vi "Unflatten U16.vi"(3 "Flat Data":u8[](array[numeric]) format="%.0x", 4 "Endian":T1) -> (5 "U16":u16)   [LabVIEW 2021, in "DataTypes_CIF_U.lvlib"]
uses:
  DataTypes_CIF_U.lvlib
  Typedef/Endian.ctl
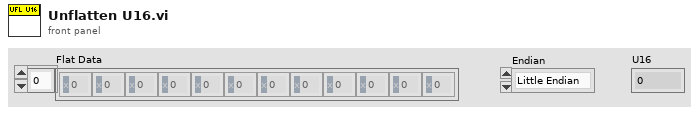
[diagram p1: front panel]
types:
  T1 = typedef "DataTypes_CIF_U.lvlib/Endian.ctl" = enum16{"Little Endian", "Big Endian"}
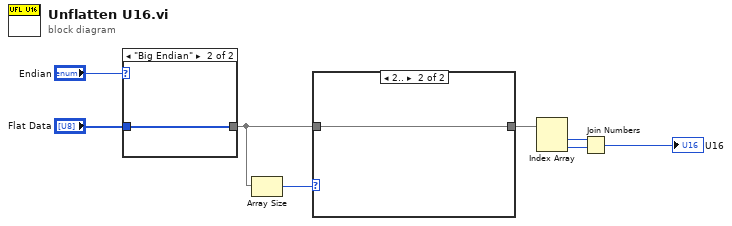
[diagram p0: block diagram]
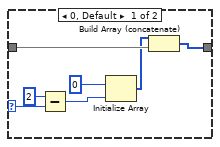
[diagram p2: hidden frame]
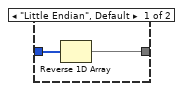
[diagram p3: hidden frame]
diagram:
  n1 = case shown="\"Big Endian\"" "Endian" {
    tunnel: "Flat Data" -> [w10 w11]
    tunnel: [w9 w11] -> w2
    frame "Little Endian", Default {
      n2 = Reverse 1D Array(array=w10) -> (reversed array=w9:u8[])
    }
    frame "Big Endian" {
    }
  }
  n3 = Array Size(array=w2) -> (size(s)=w5:i32)
  n4 = case shown="2.." w5 {
    selector: w5 -> [w18 _]
    tunnel: w2 -> [w14 w19]
    tunnel: [w12 w19] -> w3
    frame 0, Default {
      n5 = Subtract(x=2, y=w18) -> (x-y=w15:i32)
      n6 = Initialize Array(u8 0 ("element"), w15) -> (w13:u8[])
      n7 = Build Array (concatenate)(w13, w14) -> (w12:u8[])
    }
    frame 2.. {
    }
  }
  n8 = Index Array(array=w3) -> (element #1=w7:u8, element #2=w6:u8)  [unwired: 2 in]
  n9 = Join Numbers(hi=w7, lo=w6) -> ((hi.lo)=→"U16":u16)
